vi "Initialize.vi"(8 "error in (no error)":errorcluster, 10 "Device":string) -> (0 "error out":errorcluster, 3 "Temp Chamber":refnum<class "Temp Chamber.lvclass">)   [LabVIEW 2018, in "Temp Chamber.lvlib" / "Temp Chamber.lvclass"]
uses:
  Temp Chamber.lvclass
  Temp Chamber.lvclass/Temp Chamber.ctl
  PPLs/Configuration/Configuration.lvlibp/Configuration.lvclass
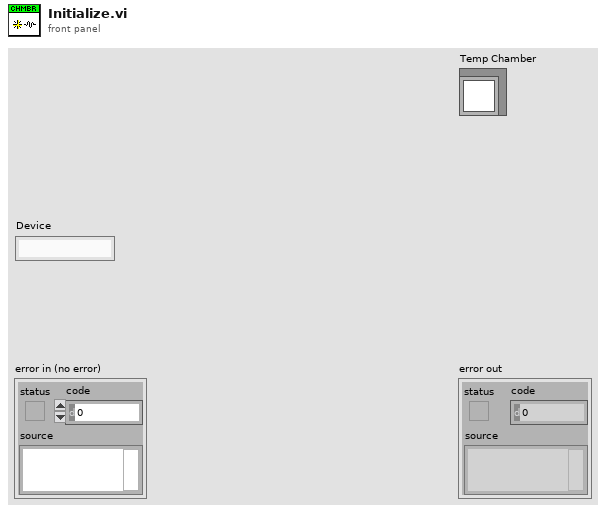
[diagram p1: front panel]
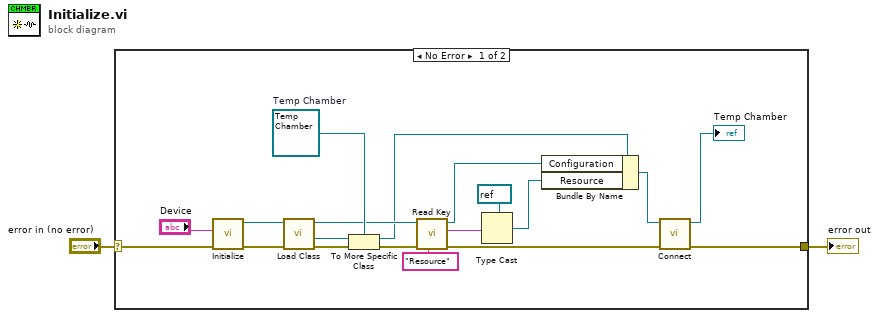
[diagram p0: block diagram]
diagram:
  n1 = case shown="No Error" "error in (no error)" {
    selector: "error in (no error)" -> [w21 w22]
    tunnel: [w8 w22] -> w1
    frame No Error {
      w16 = refnum<class "Temp Chamber.lvclass"> refnum  # Temp Chamber
      n2 = call "Initialize.vi"("error in"=w21, "Device"="Device") -> ("error out"=w18:errorcluster, "Configuration out"=w19:refnum<class "Configuration.lvclass">)  [unwired: 8 in]
      n3 = call "Load Class.vi"("error in"=w18, "Configuration in"=w19) -> ("error out"=w17:errorcluster, "Class out"=w15:refnum<class>, "Configuration out"=w13:refnum<class "Configuration.lvclass">)  [unwired: 7 in]
      n4 = To More Specific Class(target class=w16, reference=w15, error in=w17) -> (specific class reference=w12:refnum<class "Temp Chamber.lvclass">, error out=w14:errorcluster)
      n5 = call "Read Key.vi"("Key:"="Resource", "error in"=w14, "Configuration in"=w13) -> ("error out"=w10:errorcluster, "Value"=w7:string, "Configuration out"=w11:refnum<class "Configuration.lvclass">)  [unwired: 6 in]
      n6 = Type Cast(type=refnum<visa-resource-name> refnum ("Resource"), x=w7) -> (*(type *) &x=w5:refnum<visa-resource-name>)
      n7 = Bundle By Name(cluster=w12, "Configuration"=w11, "Resource"=w5) -> (w9:refnum<class "Temp Chamber.lvclass">)
      n8 = call-dynamic "Connect.vi"("error in (no error)"=w10, "Temp Chamber in"=w9) -> ("error out"=w8:errorcluster, "Temp Chamber out"=→"Temp Chamber":refnum<class "Temp Chamber.lvclass">)  [unwired: 8 in]
    }
    frame Error {
    }
  }
  "error out" <- w1
